vi "get_ref_from_control.vi"(8 "error in":errorcluster, 10 "control label":string, 11 "controls array":refnum<vi>[](array[refnum])) -> (0 "error out":errorcluster, 3 "reference out":refnum<vi>)   [LabVIEW 2019]
panel:
  out "index of element":i32
  out "all labels":string[](array[string])
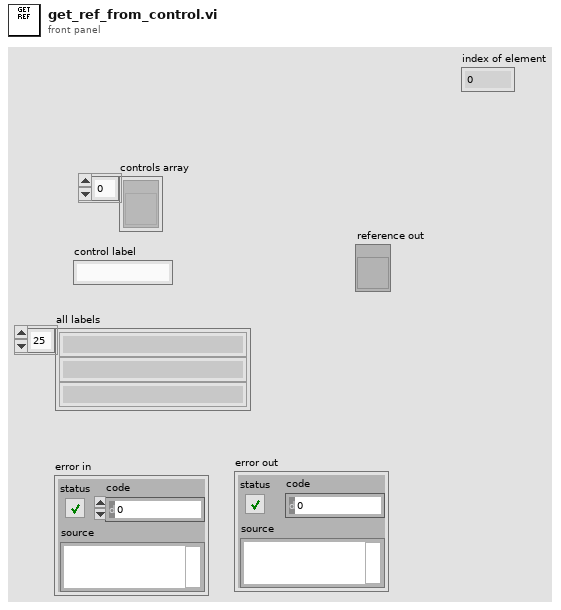
[diagram p1: front panel]
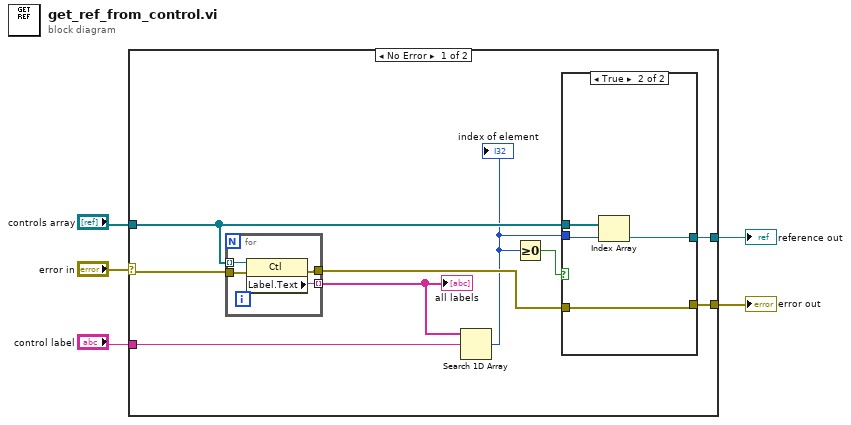
[diagram p0: block diagram]
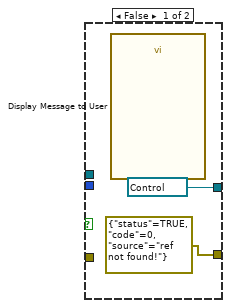
[diagram p2: hidden frame]
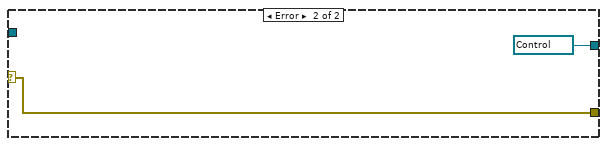
[diagram p3: hidden frame]
diagram:
  n1 = case shown="No Error" "error in" {
    selector: "error in" -> [w13 w25]
    tunnel: "control label" -> [w12 _]
    tunnel: "controls array" -> [w11 _]
    tunnel: [w9 refnum<vi> refnum ("wait after init (s)")] -> w2
    tunnel: [w7 w25] -> w1
    frame No Error {
      n2 = for {
        tunnel: w11 -> [w24] mode=indexing
        tunnel: [w23] -> w14 mode=indexing
        tunnel: w13 -> [w22]
        tunnel: [w21] -> w8
        n3 = property class="Ctl"(reference=w24, error in=w22) -> (error out=w21:errorcluster, "Label.Text"=w23:string)  [unwired: 1 out]
      }
      "all labels" <- w14
      n4 = Search 1D Array(1D array=w14, element=w12) -> (index of element=w6:i32)  [unwired: 1 in]
      "index of element" <- w6
      n5 = Greater Or Equal To 0?(x=w6) -> (x >= 0?=w10:bool)
      n6 = case shown="True" w10 {
        tunnel: w11 -> [_ w20]
        tunnel: [refnum<vi> refnum ("wait after init (s)") w19] -> w9
        tunnel: w8 -> [_ w18]
        tunnel: [errorcluster {"status"=TRUE, "code"=0, "source"="ref not found!"} ("error constant") w18] -> w7
        tunnel: w6 -> [_ w17]
        frame False {
          n7 = call "Display Message to User"() -> ()  [unwired: 10 in, 2 out]
        }
        frame True {
          n8 = Index Array(array=w20, index=w17) -> (element=w19:refnum<vi>)
        }
      }
    }
    frame Error {
    }
  }
  "reference out" <- w2
  "error out" <- w1
